vi "Read.vi"(8 "error in":errorcluster, 10 "Request Number of Message":i32=1, 11 "CanHandleIn":T1) -> (0 "error out":errorcluster, 2 "Messages":T2[](array[typedef]), 3 "CanHandleOut":T1)   [LabVIEW 2011, in "Konvolucio MCAN120803.lvlib"]
doc: "Reading a specified number of messages in the frame buffer."
uses:
  <instrlib>/Konvolucio MCAN120803/Konvolucio MCAN120803.lvlib
  <instrlib>/Konvolucio MCAN120803/Types/MessageType.ctl
  <instrlib>/Konvolucio MCAN120803/Types/CanHandleType.ctl
  C:/Program Files/National Instruments/LabVIEW 2011/instr.lib/Konvolucio MCAN120803/Private/Konvolucio.MCAN120803.API.dll
  Private/Konvolucio.MCAN120803.API.dll
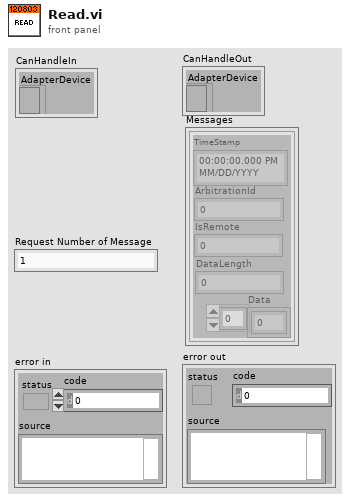
[diagram p1: front panel]
types:
  T1 = typedef "Konvolucio MCAN120803.lvlib/CanHandleType.ctl" = cluster{"AdapterDevice":refnum<k24>}
  T2 = typedef "Konvolucio MCAN120803.lvlib/MessageType.ctl" = cluster{"TimeStamp":timestamp, "ArbitrationId":u32, "IsRemote":u8, "DataLength":u8, "Data":u8[]}
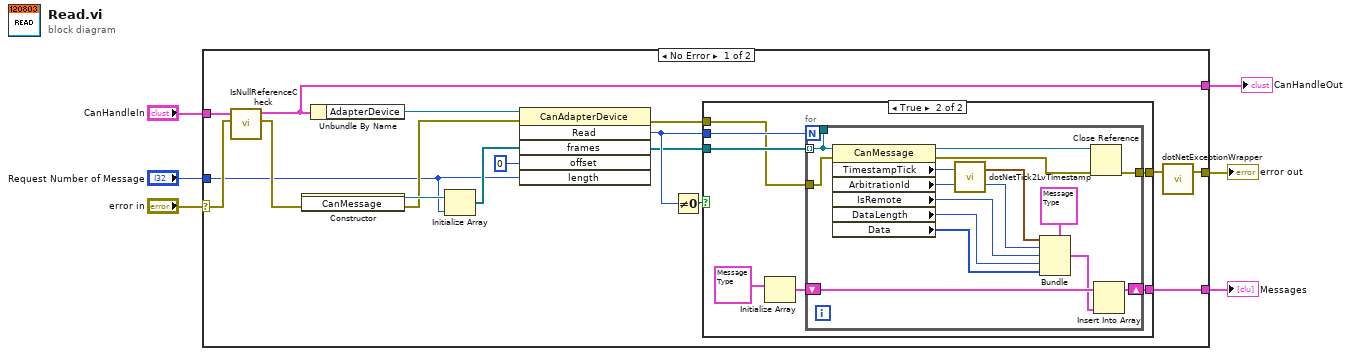
[diagram p0: block diagram]
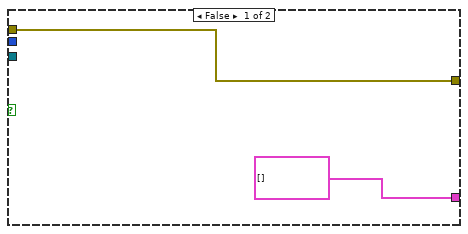
[diagram p2: hidden frame]
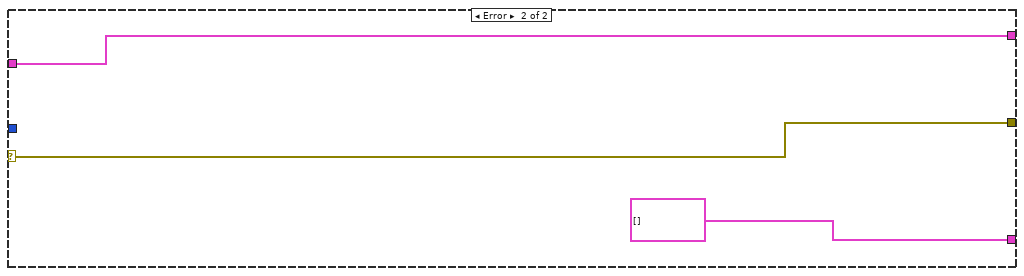
[diagram p3: hidden frame]
diagram:
  n1 = case shown="No Error" "error in" {
    selector: "error in" -> [w16 w49]
    tunnel: "Request Number of Message" -> [w12 _]
    tunnel: [w23 T2[] []] -> w5
    tunnel: [w21 w49] -> w4
    tunnel: "CanHandleIn" -> [w17 w48]
    tunnel: [w15 w48] -> w1
    frame No Error {
      n2 = call <instrlib>:"IsNullReferenceCheck.vi"("error in"=w16, "MCanHandleIn"=w17) -> ("error out"=w18:errorcluster, "MCanHandleOut"=w15:T1)  [unwired: 5 in]
      n3 = constructor class="CanMessage"(error in=w18) -> (reference out=w19:refnum<k24>, error out=w14:errorcluster)  [unwired: 2 in, 1 out]
      n4 = Unbundle By Name(w15) -> ("AdapterDevice"=w7:refnum<k24>)
      n5 = Initialize Array(w19, w12) -> (w13:refnum<k24>[])
      n6 = invoke class="CanAdapterDevice" method="Read"(reference=w7, error in=w14, "frames"=w13, "offset"=0, "length"=w12) -> (error out=w10:errorcluster, "Read"=w9:i32, "frames"=w8:refnum<k24>[])  [unwired: 1 in, 3 out]
      n7 = Not Equal To 0?(x=w9) -> (x != 0?=w22:bool)
      n8 = case shown="True" w22 {
        tunnel: w9 -> [_ w31]
        tunnel: w8 -> [_ w29]
        tunnel: w10 -> [w25 w28]
        tunnel: [T2[] [] w27] -> w23
        tunnel: [w25 w26] -> w20
        frame False {
        }
        frame True {
          n9 = Initialize Array(T2 {"TimeStamp"=timestamp(0 s since 1904-01-01), "ArbitrationId"=0, "IsRemote"=0, "DataLength"=0, "Data"=[]}) -> (w30:T2[])  [unwired: 1 in]
          n10 = for {
            N: w31 -> [_]
            tunnel: w29 -> [w33] mode=indexing
            tunnel: w28 -> [w43]
            shift-right: [w45] -> w27
            shift-left: w30 -> [w47]
            tunnel: [w44] -> w26
            tunnel: [w33] -> _
            n11 = property class="CanMessage"(reference=w33, error in=w43) -> (reference out=w42:refnum<k24>, error out=w41:errorcluster, "TimestampTick"=w39:i64, "ArbitrationId"=w37:u32, "IsRemote"=w36:u8, "DataLength"=w35:u8, "Data"=w34:u8[])
            n12 = call <instrlib>:"dotNetTick2LvTimestamp.vi"(".NetTick"=w39) -> ("time stamp"=w38:timestamp)  [unwired: 2 in]
            n13 = Bundle(cluster=T2 {"TimeStamp"=timestamp(0 s since 1904-01-01), "ArbitrationId"=0, "IsRemote"=0, "DataLength"=0, "Data"=[]}, "TimeStamp"=w38, "ArbitrationId"=w37, "IsRemote"=w36, "DataLength"=w35, "Data"=w34) -> (w46:T2)
            n14 = Close Reference(reference=w42, error in (no error)=w41) -> (error out=w44:errorcluster)
            n15 = Insert Into Array(array=w47, new element=w46) -> (w45:T2[])  [unwired: 1 in]
          }
        }
      }
      n16 = call <instrlib>:"dotNetExceptionWrapper.vi"("error in"=w20) -> ("error out"=w21:errorcluster)  [unwired: 2 in]
    }
    frame Error {
    }
  }
  "error out" <- w4
  "Messages" <- w5
  "CanHandleOut" <- w1
